vi "Termometr_color.vi"(2 "Temperature":dbl) -> (7 "Scale color":u32(colorbox))   [LabVIEW 2012]
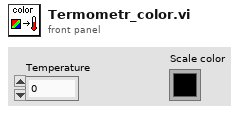
[diagram p1: front panel]
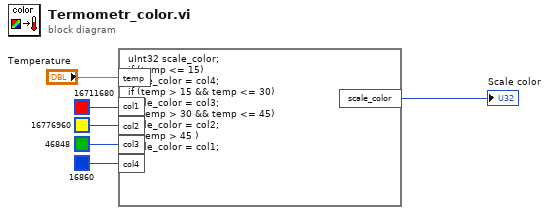
[diagram p0: block diagram]
diagram:
  n1 = formula code="uInt32 scale_color;\nif (temp <= 15)\nscale_color = col4;\nif (temp > 15 && temp <= 30)\nscale_color = col3;\nif (temp > 30 && temp <= 45)\nscale_color = col2;\nif (temp > 45 )\nscale_color = col1;"("temp"="Temperature", "col1"=u32 16711680, "col2"=u32 16776960, "col3"=u32 46848, "col4"=u32 16860) -> ("scale_color"=→"Scale color":u32)
